vi "tlc_Initialize.vi"(7 "Number of Channels":cluster{"Rows":i32, "Columns":i32}, 8 "error in (no error)":errorcluster, 9 "tlc_Consumer Queue Reference.ctl":T1, 10 "tlc_Display Queue Reference.ctl":T2, 11 "tlc_User Event Reference.ctl":T3) -> (0 "error out":errorcluster)   [LabVIEW 2009]
doc: "[Covers: REQ_Initialize]\nThis VI initializes the system."
uses:
  Controls/tlc_User Event Reference.ctl
  Controls/tlc_Display Queue Reference.ctl
  Controls/tlc_User Interface Command.ctl
  Controls/tlc_User Interface Data Type.ctl
  Controls/tlc_Consumer Queue Reference.ctl
  Controls/tlc_Consumer Control.ctl
  Controls/tlc_Functions.ctl
  Modules/Hardware/tlc_Hardware_Command Control.ctl
  Modules/File/tlc_File_Command Control.ctl
  Modules/Cue/tlc_Cue_Information Command.ctl
  Modules/Error/tlc_Error Module Command Control.ctl
  Modules/Display/tlc_Display_Command Control.ctl
panel:
  # "Input"
  # "Output"
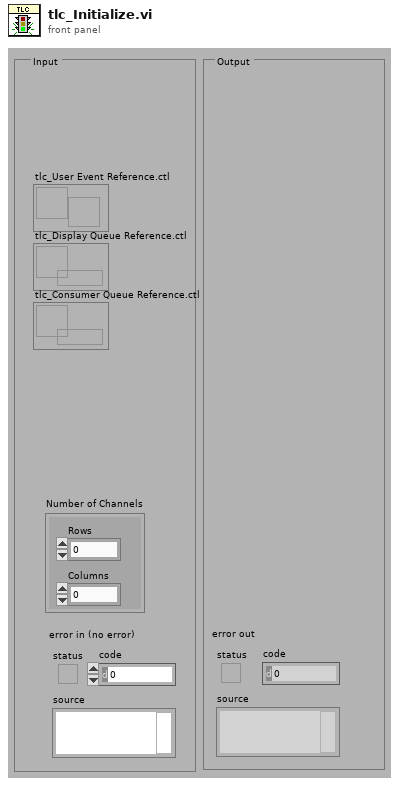
[diagram p1: front panel]
types:
  T1 = typedef "tlc_Consumer Queue Reference.ctl" = refnum<queue>
  T2 = typedef "tlc_Display Queue Reference.ctl" = refnum<queue>
  T3 = typedef "tlc_User Event Reference.ctl" = refnum<user-event>
  T4 = typedef "tlc_User Interface Data Type.ctl" = enum16{"Initialize", "Initialize Front Panel", "Update Front Panel Channels", "Select Cue in Cue List", "Enable/Disable Front Panel Controls", "Update Cue List", "Stop"}
  T5 = typedef "tlc_Hardware_Command Control.ctl" = enum16{"Initialize", "Write", "Shutdown"}
  T6 = typedef "tlc_File_Command Control.ctl" = enum16{"Initialize", "Save Cues", "Load Cues", "Shutdown"}
  T7 = typedef "tlc_Cue_Information Command.ctl" = enum16{"Add Cue", "Get Cue Values", "Set Cue Values", "Get Number of Cues", "Initialize", "Get Empty Cue"}
  T8 = typedef "tlc_Error Module Command Control.ctl" = enum16{"Initialize", "Handle Errors", "Report Errors"}
  T9 = typedef "tlc_Display_Command Control.ctl" = enum16{"Initialize", "Update UI", "Shutdown"}
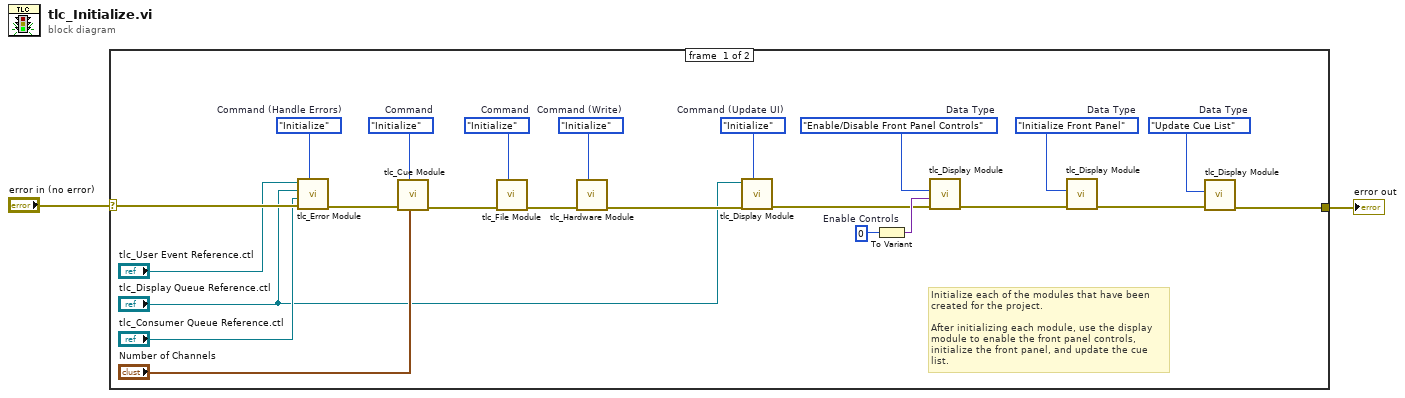
[diagram p0: block diagram]
diagram:
  n1 = case shown="No Error" "error in (no error)" {
    selector: "error in (no error)" -> [w25 w26]
    tunnel: [w11 w26] -> w1
    frame #0 {
      w8 = i8 0  # Enable Controls
      w10 = tlc_User_Interface_Data_Type."Update Cue List"  # Data Type
      w13 = tlc_User_Interface_Data_Type."Initialize Front Panel"  # Data Type
      w15 = tlc_User_Interface_Data_Type."Enable/Disable Front Panel Controls"  # Data Type
      w16 = tlc_Hardware_Command_Control."Initialize"  # Command (Write)
      w18 = tlc_File_Command_Control."Initialize"  # Command
      w20 = tlc_Cue_Information_Command."Initialize"  # Command
      w21 = tlc_Error_Module_Command_Control."Initialize"  # Command (Handle Errors)
      w22 = tlc_Display_Command_Control."Initialize"  # Command (Update UI)
      # "Initialize each of the modules that have been created for the project.\n\nAfter initializing each module, use the display module to enable the front panel controls, initialize the front panel, and update the cue list."
      n2 = call "tlc_Error Module.vi"("Command (Handle Errors"=w21, "error in (no error)"=w25, "tlc_Consumer Queue Reference.ctl"="tlc_Consumer Queue Reference.ctl", "tlc_Display Queue Reference.ctl"="tlc_Display Queue Reference.ctl", "tlc_User Event Reference.ctl"="tlc_User Event Reference.ctl") -> ("error out"=w6:errorcluster)  [unwired: 5 in, 1 out]
      n3 = call "tlc_Cue Module.vi"("Number of Channels"="Number of Channels", "Command"=w20, "error in (no error)"=w6) -> ("error out"=w19:errorcluster)  [unwired: 5 in, 2 out]
      n4 = call "tlc_File Module.vi"("Command"=w18, "error in (no error)"=w19) -> ("error out"=w17:errorcluster)  [unwired: 8 in, 1 out]
      n5 = call "tlc_Hardware Module.vi"("Command (Write)"=w16, "error in (no error)"=w17) -> ("error out"=w5:errorcluster)  [unwired: 9 in]
      n6 = call "tlc_Display Module.vi"("Command (Update UI)"=w22, "error in (no error)"=w5, "tlc_Display Queue Reference.ctl"="tlc_Display Queue Reference.ctl") -> ("error out"=w4:errorcluster)  [unwired: 8 in]
      n7 = To Variant(anything=w8) -> (Variant=w7:variant)
      n8 = call "tlc_Display Module.vi"("error in (no error)"=w4, "Data"=w7, "Data Type"=w15) -> ("error out"=w14:errorcluster)  [unwired: 8 in]
      n9 = call "tlc_Display Module.vi"("error in (no error)"=w14, "Data Type"=w13) -> ("error out"=w12:errorcluster)  [unwired: 9 in]
      n10 = call "tlc_Display Module.vi"("error in (no error)"=w12, "Data Type"=w10) -> ("error out"=w11:errorcluster)  [unwired: 9 in]
    }
    frame #1 {
    }
  }
  "error out" <- w1
